vi "Rename & Move Entire Library.vi"(0 "Application":refnum<vi>, 1 "New Name Without Extension":string, 5 "Library Path":path, 9 "Project":refnum<vi>, 11 "error in":errorcluster, 14 "Rename File only(T)":bool) -> (4 "Application out":refnum<vi>, 6 "New Library Path":path, 15 "error out":errorcluster)   [LabVIEW 2020, in "PluginMetaDataObj.lvclass"]
doc: "This VI either renames the file name alone or renames both the file name and folder name"
uses:
  PluginMetaDataObj.lvclass
  <vilib>/Utility/EditLVLibs/Edit LVLibs.lvlib
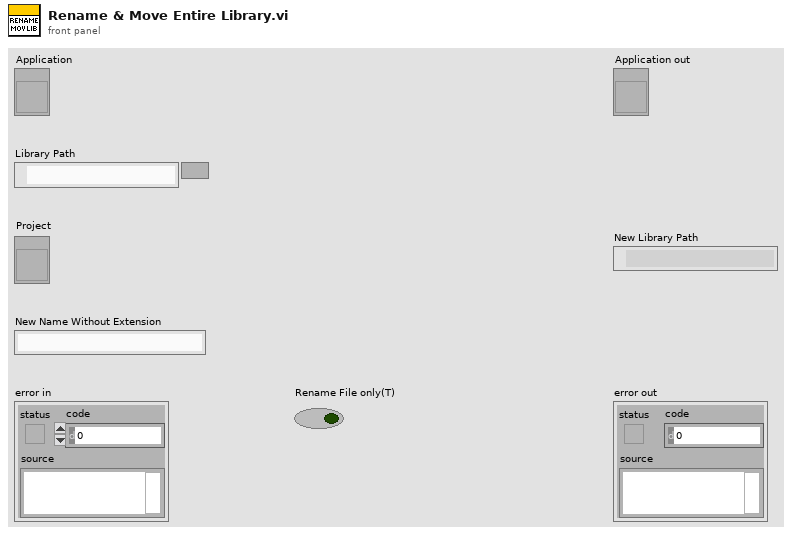
[diagram p1: front panel]
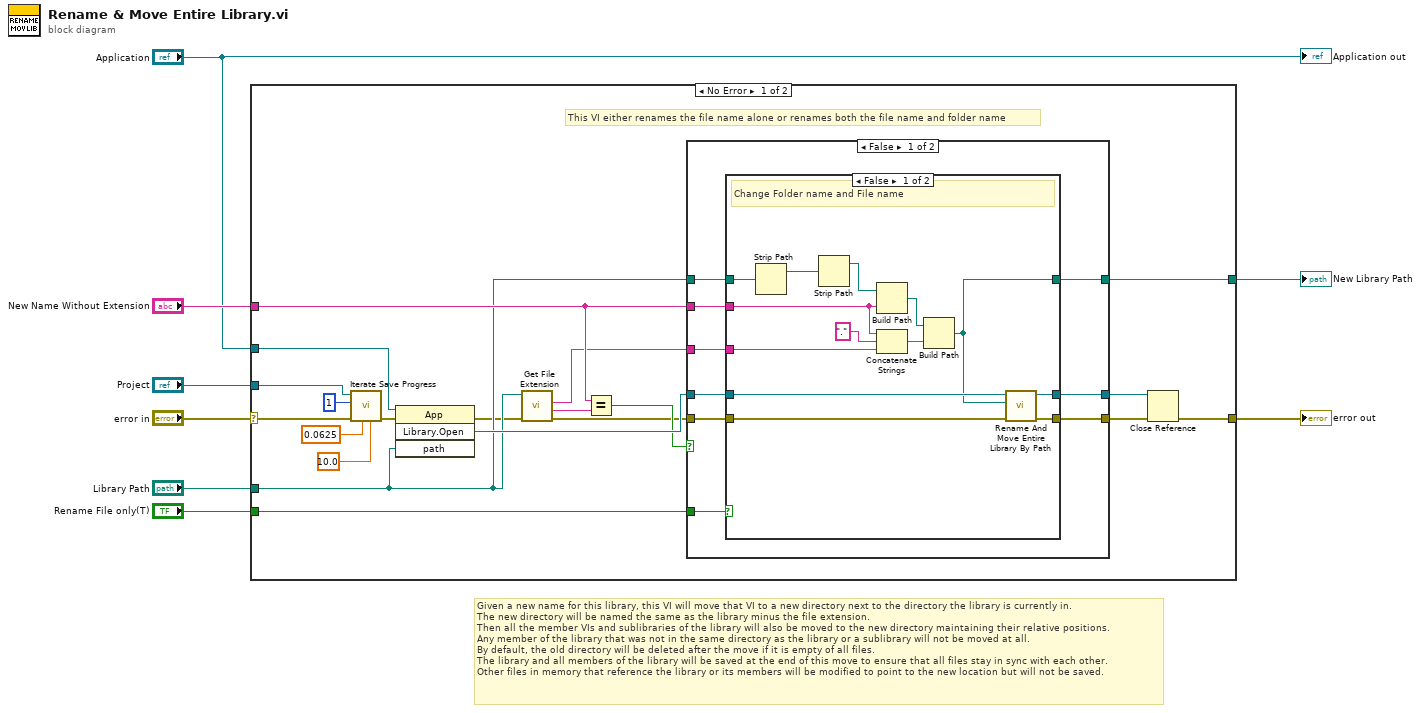
[diagram p0: block diagram]
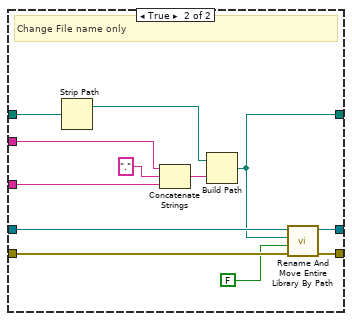
[diagram p2: hidden frame]
diagram:
  # "Given a new name for this library, this VI will move that VI to a new directory next to the directory the library is currently in. \nThe new directory will be named the same as the library minus the file extension. \nThen all the member VIs and sublibraries of the library will also be moved to the new directory maintaining their relative positions. \nAny member of the library that was not in the same directory as the library or a sublibrary will not be moved at all. \nBy default, the old directory will be deleted after the move if it is empty of all files. \nThe library and all members of the library will be saved at the end of this move to ensure that all files stay in sync with each other. \nOther files in memory that reference the library or its members will be modified to point to the new location but will not be saved."
  n1 = case shown="No Error" "error in" {
    selector: "error in" -> [w23 w66]
    tunnel: "Application" -> [w28 _]
    tunnel: "Library Path" -> [w11 _]
    tunnel: "New Name Without Extension" -> [w20 _]
    tunnel: [w17 _] -> w6
    tunnel: [w27 w66] -> w5
    tunnel: "Project" -> [w21 _]
    tunnel: "Rename File only(T)" -> [w18 _]
    frame No Error {
      # "This VI either renames the file name alone or renames both the file name and folder name"
      n2 = call <resource>:"Iterate Save Progress.vi"("Total Iteration Progress"=10.0 ("This Task's Percentage"), "This Task's Percentage"=0.0625, "error in (no error)"=w23, "Total Iterations (this task)"=1, "Project"=w21) -> ("error out"=w22:errorcluster)  [unwired: 6 in]
      n3 = invoke class="App" method="Library.Open"(reference=w28, error in=w22, "path"=w11) -> (error out=w10:errorcluster, "Open Library"=w19:refnum<vi>)  [unwired: 1 in, 2 out]
      n4 = call <vilib>:"Get File Extension.vi"("error in (no error)"=w10, "file"=w11) -> ("error out"=w9:errorcluster, "filename without extension"=w13:string, "lowercase file extension"=w12:string)  [unwired: 5 in, 2 out]
      n5 = Equal?(x=w20, y=w13) -> (x = y?=w14:bool)
      n6 = case shown="False" w14 {
        tunnel: w20 -> [w36 _]
        tunnel: [w37 w65] -> w15
        tunnel: w9 -> [w33 w65]
        tunnel: [w35 w64] -> w16
        tunnel: w19 -> [w34 w64]
        tunnel: w11 -> [w32 w63]
        tunnel: w12 -> [w31 _]
        tunnel: [w30 w63] -> w17
        tunnel: w18 -> [w29 _]
        frame False {
          n7 = case shown="False" w29 {
            tunnel: [w50 w62] -> w37
            tunnel: w36 -> [w46 w60]
            tunnel: [w44 w58] -> w35
            tunnel: w34 -> [w43 w57]
            tunnel: w33 -> [w42 w56]
            tunnel: w32 -> [w40 w54]
            tunnel: w31 -> [w39 w53]
            tunnel: [w38 w52] -> w30
            frame False {
              # "Change Folder name and File name"
              n8 = Strip Path(path=w40) -> (stripped path=w41:path)  [unwired: 1 out]
              n9 = Strip Path(path=w41) -> (stripped path=w49:path)  [unwired: 1 out]
              n10 = Build Path(base path=w49, name or relative path=w46) -> (appended path=w48:path)
              n11 = Concatenate Strings(w46, "." ("string"), w39) -> (w45:string)
              n12 = Build Path(base path=w48, name or relative path=w45) -> (appended path=w38:path)
              n13 = call <vilib>:"Rename And Move Entire Library By Path.vi"("error in (no error)"=w42, "New library path"=w38, "Library ref in"=w43) -> ("error out"=w50:errorcluster, "Library ref out"=w44:refnum<vi>)  [unwired: 7 in]
            }
            frame True {
              # "Change File name only"
              n14 = Strip Path(path=w54) -> (stripped path=w55:path)  [unwired: 1 out]
              n15 = Concatenate Strings(w60, "." ("string"), w53) -> (w59:string)
              n16 = Build Path(base path=w55, name or relative path=w59) -> (appended path=w52:path)
              n17 = call <vilib>:"Rename And Move Entire Library By Path.vi"("error in (no error)"=w56, "Delete old directory if empty after move? (T)"=FALSE, "New library path"=w52, "Library ref in"=w57) -> ("error out"=w62:errorcluster, "Library ref out"=w58:refnum<vi>)  [unwired: 6 in]
            }
          }
        }
        frame True {
        }
      }
      n18 = Close Reference(reference=w16, error in (no error)=w15) -> (error out=w27:errorcluster)
    }
    frame Error {
    }
  }
  "error out" <- w5
  "New Library Path" <- w6
  "Application out" <- "Application"
